vi "Variant Tools Test Arrays.vi"() -> ()   [LabVIEW 2013]
uses:
  <vilib>/addons/JSON API/JSON Value/JSON Value.lvclass
  <vilib>/addons/JSON API/JSON Value/Set from JSON string.vi
  <vilib>/addons/JSON API/Variant JSON/Get as Variant.vi
  JSONtext.lvlib
  <vilib>/gmath/NI_Gmath.lvlib
  <vilib>/addons/JSON API/Get Polymorphic/JSON GetSet.lvlib
  <vilib>/addons/JSON API/Variant JSON/Variant JSON.lvlib
panel:
  out "x = y?":bool
  in  "Pretty Print?":bool=TRUE
  out "Cluster 2":T1={"DBL"=[1.23456, 1.23456, 1.23456, 1.23456, 1.23456, 1.23456, 1.23456, 1.23456, 1.23456, 1.23456, 1.23456, 1.23456, 2.23456], "DBL 2"=[[1.23, 1.23, 1.23, 1.23, 1.23, 1.23, 1.23, 1.23, 1.23, 1.23, 1.23, 1.23, 1.23, 1.23, 1.23, 1.23, 1.23, 1.23, 1.23, 1.23, 1.23, 1.23, 1.23, 1.23, 1.23, 1.23, 1.23, 1.23, 1.23, 1.23, 1.23, 1.23, 1.23, 1.23, 1.23, 1.23, 1.23, 1.23, 1.23, 1.23, 1.23, 1.23, 1.23, 1.23, 1.23, 1.23, 1.23, 1.23, 1.23, 1.23, 1.23, 1.23, 1.23, 1.23, 1.23, 1.23, 1.23, 1.23, 1.23, 1.23, 1.23, 1.23, 1.23, 1.23, 1.23, 1.23, 1.23, 1.23, 1.23, 1.23, 1.23, 1.23, 1.23, 1.23, 1.23, 1.23, 1.23, 1.23, 1.23, 1.23, 1.23, 1.23, 1.23, 1.23, 1.23, 1.23, 1.23, 1.23, 1.23, 1.23, 1.23, 1.23, 1.23, 1.23, 1.23, 1.23, 1.23, 1.23, 1.23, 1.23, 2.23]], "String"=["", "", "", "", "", "", "", "", "", "", "", "", "", "", "", "", "", "", "", "", "", "", "", "", "", "", "", "", "", "", "", "", "", "", "", "", "", "", "", "", "", "", "", "", "", "", "", "", "", "", "", "", "", "", "", "", "", "", "", "", "", "", "", "", "", "", "", "", "", "", "", "", "", "", "", "", "", "", "", "", "", "", "", "", "", "", "", "", "", "", "", "", "", "", "", "", "", "", "", "", ""], "String 2"=[["", "", "", "", "", "", "", "", "", "", "", "", "", "", "", "", "", "", "", "", "", "", "", "", "", "", "", "", "", "", "", "", "", "", "", "", "", "", "", "", "", "", "", "", "", "", "", "", "", "", "", "", "", "", "", "", "", "", "", "", "", "", "", "", "", "", "", "", "", "", "", "", "", "", "", "", "", "", "", "", "", "", "", "", "", "", "", "", "", "", "", "", "", "", "", "", "", "", "", "", ""]], "<JSON>json"=[], "<JSON>json 2"=[], "I32"=[1, 1, 1, 1, 1, 1, 1, 1, 1, 1, 1, 1, 1, 1, 1, 1, 1, 1, 1, 1, 1, 1, 1, 1, 1, 1, 1, 1, 1, 1, 1, 1, 1, 1, 1, 1, 1, 1, 1, 1, 1, 1, 1, 1, 1, 1, 1, 1, 1, 1, 1, 1, 1, 1, 1, 1, 1, 1, 1, 1, 1, 1, 1, 1, 1, 1, 1, 1, 1, 1, 1, 1, 1, 1, 1, 1, 1, 1, 1, 1, 1, 1, 1, 1, 1, 1, 1, 1, 1, 1, 1, 1, 1, 1, 1, 1, 1, 1, 1, 1, 2], "Paths"=[path "C:/", path ""]}
  in  "Old JSON":bool
  out "mean":dbl format="%.3p"
  out "Variant out":variant
  out "To Variant":dbl[](array[numeric]) format="%#_3p"
  in  "Cluster":T1={"DBL"=[inf, -inf, 1.23, 1.23, 1.23, 1.23, 1.23, 1.23, 1.23, 1.23, 1.23, 1.23, 1.23, 1.23, 1.23, 1.23, 1.23, 1.23, 1.23, 1.23, 1.23, 1.23, 1.23, 1.23, 1.23, 1.23, 1.23, 1.23, 1.23, 1.23, 1.23, 1.23, 1.23, 1.23, 1.23, 1.23, 1.23, 1.23, 1.23, 1.23, 1.23, 1.23, 1.23, 1.23, 1.23, 1.23, 1.23, 1.23, 1.23, 1.23, 1.23, 1.23, 1.23, 1.23, 1.23, 1.23, 1.23, 1.23, 1.23, 1.23, 1.23, 1.23, 1.23, 1.23, 1.23, 1.23, 1.23, 1.23, 1.23, 1.23, 1.23, 1.23, 1.23, 1.23, 1.23, 1.23, 1.23, 1.23, 1.23, 1.23, 1.23, 1.23, 1.23, 1.23, 1.23, 1.23, 1.23, 1.23, 1.23, 1.23, 1.23, 1.23, 1.23, 1.23, 1.23, 1.23, 1.23, 1.23, 1.23, 1.23, 2.23], "DBL 2"=[[1.23, 1.23, 1.23, 1.23, 1.23, 1.23, 1.23, 1.23, 1.23, 1.23, 1.23, 1.23, 1.23, 1.23, 1.23, 1.23, 1.23, 1.23, 1.23, 1.23, 1.23, 1.23, 1.23, 1.23, 1.23, 1.23, 1.23, 1.23, 1.23, 1.23, 1.23, 1.23, 1.23, 1.23, 1.23, 1.23, 1.23, 1.23, 1.23, 1.23, 1.23, 1.23, 1.23, 1.23, 1.23, 1.23, 1.23, 1.23, 1.23, 1.23, 1.23, 1.23, 1.23, 1.23, 1.23, 1.23, 1.23, 1.23, 1.23, 1.23, 1.23, 1.23, 1.23, 1.23, 1.23, 1.23, 1.23, 1.23, 1.23, 1.23, 1.23, 1.23, 1.23, 1.23, 1.23, 1.23, 1.23, 1.23, 1.23, 1.23, 1.23, 1.23, 1.23, 1.23, 1.23, 1.23, 1.23, 1.23, 1.23, 1.23, 1.23, 1.23, 1.23, 1.23, 1.23, 1.23, 1.23, 1.23, 1.23, 1.23, 2.23, inf]], "String"=["one", "zero\u0000char"], "String 2"=[["one", "two"], ["three", "zero\u0000char"]], "<JSON>json"=["\"my_json\"", "123456.789", "\"longgggggggg string\""], "<JSON>json 2"=[["\"my_json\"", "123456.789", "\"longgggggggg string\""], ["\"A\"", "123", "345"]], "I32"=[1, 1, 1, 1, 1, 1, 1, 1, 1, 1, 1, 1, 1, 1, 1, 1, 1, 1, 1, 1, 1, 1, 1, 1, 1, 1, 1, 1, 1, 1, 1, 1, 1, 1, 1, 1, 1, 1, 1, 1, 1, 1, 1, 1, 1, 1, 1, 1, 1, 1, 1, 1, 1, 1, 1, 1, 1, 1, 1, 1, 1, 1, 1, 1, 1, 1, 1, 1, 1, 1, 1, 1, 1, 1, 1, 1, 1, 1, 1, 1, 1, 1, 1, 1, 1, 1, 1, 1, 1, 1, 1, 1, 1, 1, 1, 1, 1, 1, 1, 1, 2], "Paths"=[path "C:/", path "abc"]}
  out "<JSON>":string
  out "error out":errorcluster
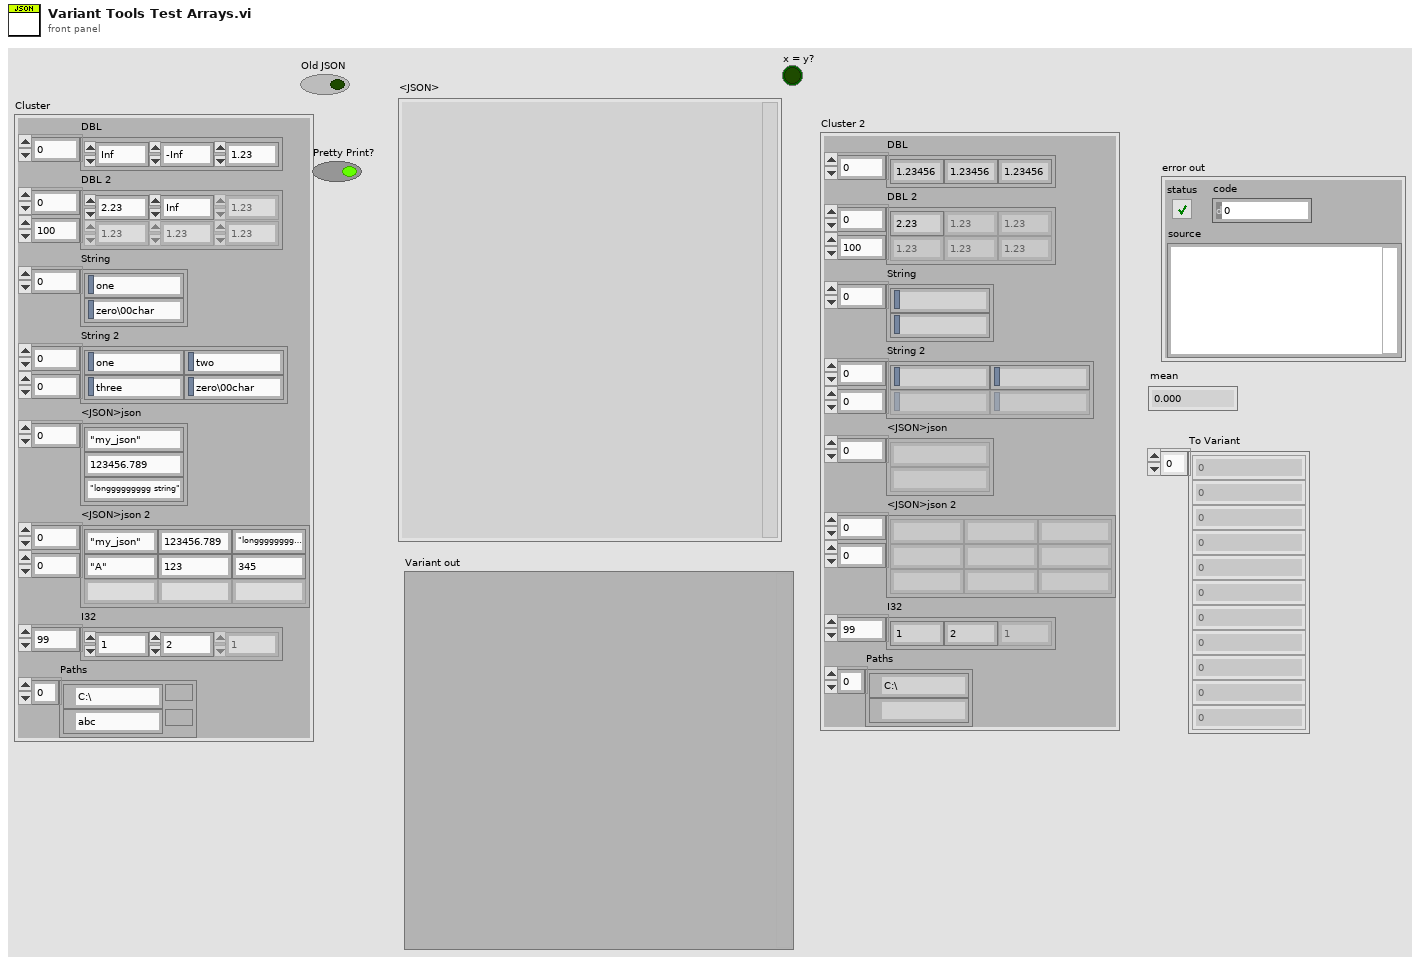
[diagram p1: front panel]
types:
  T1 = cluster{"DBL":dbl[], "DBL 2":dbl[][], "String":string[], "String 2":string[][], "<JSON>json":string[], "<JSON>json 2":string[][], "I32":i32[], "Paths":path[]}
  T2 = enum16{"arithmetic", "geometric", "harmonic", "trimmed", "median"}
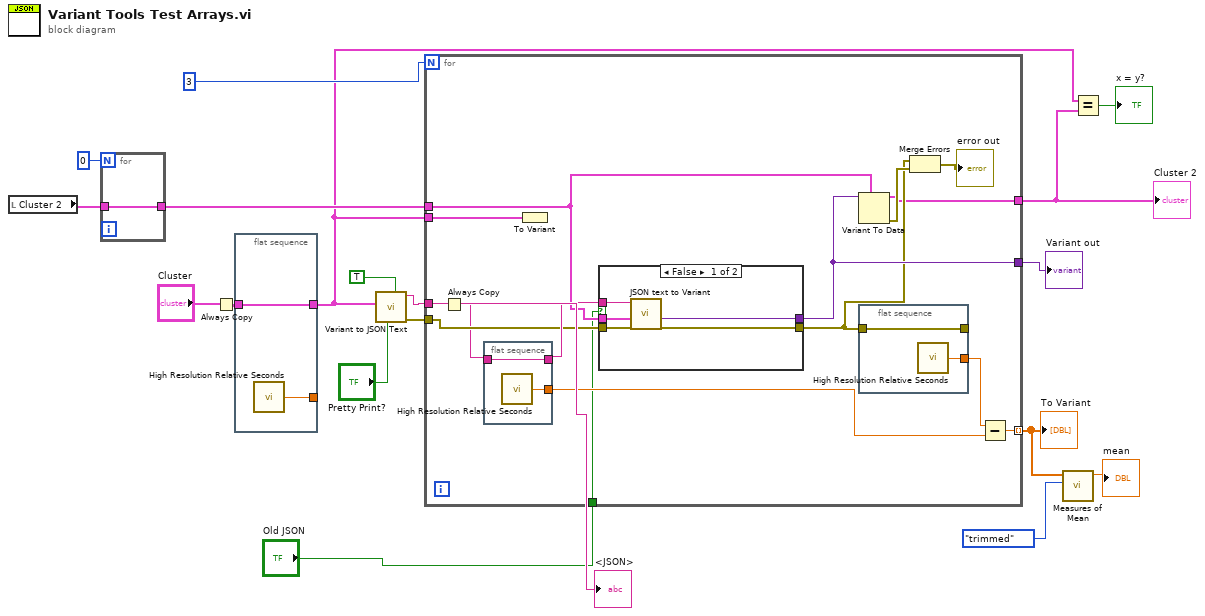
[diagram p0: block diagram]
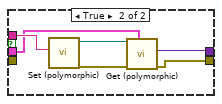
[diagram p2: hidden frame]
diagram:
  n1 = local read "Cluster 2"() -> (w15:T1)
  n2 = for {
    N: 0 -> [_]
    tunnel: [w19] -> w16
    tunnel: w15 -> [w19]
  }
  n3 = Always Copy(1:"Cluster") -> (0:w10:T1)
  n4 = flat-sequence {
    tunnel: w10 -> [w20]
    tunnel: [w21] -> _
    tunnel: [w20] -> w3
    frame #0 {
      n5 = call <vilib>:"High Resolution Relative Seconds.vi"() -> ("relative seconds"=w21:dbl)
    }
  }
  n6 = call "Variant to JSON Text.vi"("enable LabVIEW extensions? (T)"=TRUE, "Pretty Print?"="Pretty Print?", "Variant"=w3) -> ("error out"=w11:errorcluster, "<JSON>"=w8:string)  [unwired: 7 in]
  "<JSON>" <- w8
  n7 = for {
    N: 3 -> [_]
    tunnel: [w36] -> w6 mode=indexing
    tunnel: w16 -> [w35]
    tunnel: w8 -> [w27]
    tunnel: [w22] -> w2
    tunnel: [w34] -> w14
    tunnel: w3 -> [w31]
    tunnel: w11 -> [w25]
    tunnel: "Old JSON" -> [w23]
    n8 = Always Copy(1:w27) -> (0:w24:string)
    n9 = flat-sequence {
      tunnel: [w49] -> w26
      tunnel: w24 -> [w49]
      tunnel: [w48] -> w30
      frame #0 {
        n10 = call <vilib>:"High Resolution Relative Seconds.vi"() -> ("relative seconds"=w48:dbl)
      }
    }
    n11 = To Variant(anything=w31) -> ()  [unwired: 1 out]
    n12 = case shown="False" w23 {
      tunnel: w35 -> [w41 w46]
      tunnel: [w40 w44] -> w34
      tunnel: [w39 w43] -> w28
      tunnel: w26 -> [w38 w47]
      tunnel: w25 -> [w37 _]
      frame False {
        n13 = call "JSON text to Variant.vi"("error in (no error)"=w37, "Data Type"=w41, "JSON"=w38) -> ("error out"=w39:errorcluster, "Variant out"=w40:variant)  [unwired: 7 in]
      }
      frame True {
        n14 = call-poly <vilib>:"Set (polymorphic).vi"("JSON stream"=w47) -> ("error out"=w42:errorcluster, "JSON Value out"=w45:refnum<class "JSON Value.lvclass">)  [unwired: 8 in, 1 out]
        n15 = call-poly <vilib>:"Get (polymorphic).vi"("Variant (Data Type)"=w46, "error in (no error)"=w42, "JSON in"=w45) -> ("error out"=w43:errorcluster, "Variant out"=w44:variant)  [unwired: 6 in, 1 out]
      }
    }
    n16 = Variant To Data(type=w35, Variant=w34) -> (data=w22:T1, error out=w33:errorcluster)  [unwired: 1 in]
    n17 = flat-sequence {
      tunnel: [w51] -> _
      tunnel: w28 -> [w51]
      tunnel: [w50] -> w32
      frame #0 {
        n18 = call <vilib>:"High Resolution Relative Seconds.vi"() -> ("relative seconds"=w50:dbl)
      }
    }
    n19 = Merge Errors(w28, w33) -> (→"error out":errorcluster)
    n20 = Subtract(x=w32, y=w30) -> (x-y=w36:dbl)
  }
  "To Variant" <- w6
  "Variant out" <- w14
  "Cluster 2" <- w2
  n21 = call <vilib>:"Measures of Mean.vi"("type"=T2."trimmed", "x array"=w6) -> ("mean value"=→"mean":dbl)  [unwired: 8 in, 1 out]
  n22 = Equal?(x=w3, y=w2) -> (x = y?=→"x = y?":bool)
